vi "Pts_Plot (SubVI).vi"(10 "Ref WF":dbl[](array[numeric]), 11 "Locations":dbl[](array[numeric])) -> (3 "Waveform":dbl[](array[numeric]))   [LabVIEW 2017]
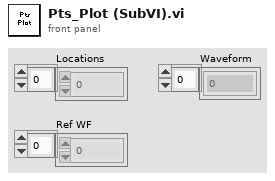
[diagram p1: front panel]
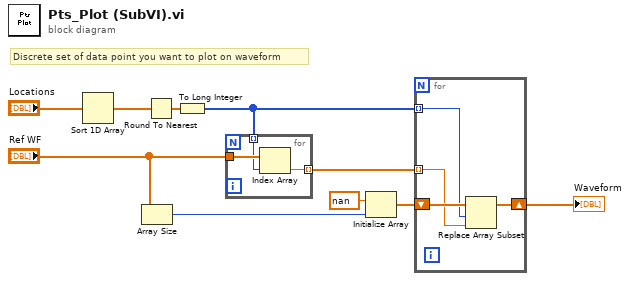
[diagram p0: block diagram]
diagram:
  # "Discrete set of data point you want to plot on waveform"
  n1 = Sort 1D Array(array="Locations") -> (sorted array=w1:dbl[])
  n2 = Array Size(array="Ref WF") -> (size(s)=w6:i32)
  n3 = Round To Nearest(number=w1) -> (nearest integer value=w9:dbl[])
  n4 = To Long Integer(number=w9) -> (32bit integer=w4:i32[])
  n5 = for {
    tunnel: "Ref WF" -> [w13]
    tunnel: w4 -> [w12] mode=indexing
    tunnel: [w11] -> w3 mode=indexing
    n6 = Index Array(array=w13, index=w12) -> (element=w11:dbl)
  }
  n7 = Initialize Array(nan ("element"), w6) -> (w7:dbl[])
  n8 = for {
    tunnel: w4 -> [w14] mode=indexing
    shift-right: [w15] -> w10
    shift-left: w7 -> [w17]
    tunnel: w3 -> [w16] mode=indexing
    n9 = Replace Array Subset(array=w17, new element=w16, index=w14) -> (w15:dbl[])
  }
  "Waveform" <- w10
